vi "RadiansToDegrees.vi"(1 "Radians":dbl) -> (0 "Degrees":dbl)   [LabVIEW 2016]
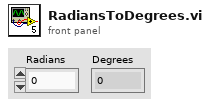
[diagram p1: front panel]
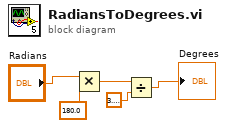
[diagram p0: block diagram]
diagram:
  n1 = Multiply(x="Radians", y=180.0) -> (x*y=w2:dbl)
  n2 = Divide(x=w2, y=3.141592653589793) -> (x/y=→"Degrees":dbl)
